vi "cmd.vi"(5 "value format":string="%g", 7 "template":string="SOUR<channel>:VOLT:HIGH <value>", 10 "channel":string="1", 11 "value":dbl) -> (2 "cmd":string="SOUR1:VOLT:HIGH 0.000000")   [LabVIEW 2017, in "serial.lvlib"]
uses:
  serial.lvlib
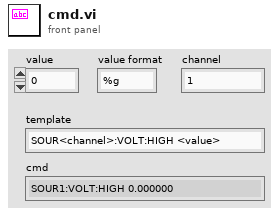
[diagram p1: front panel]
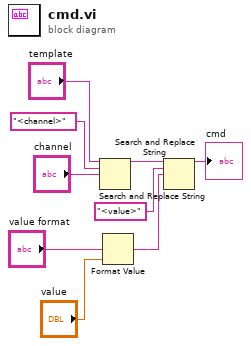
[diagram p0: block diagram]
diagram:
  n1 = Search and Replace String(input string="template", search string="<channel>", replace string="channel") -> (result string=w3:string)  [unwired: 5 in, 3 out]
  n2 = Format Value(format string="value format", value (0)="value") -> (output string=w2:string)  [unwired: 1 in]
  n3 = Search and Replace String(input string=w3, search string="<value>", replace string=w2) -> (result string=→"cmd":string)  [unwired: 5 in, 3 out]
